vi "Get Column Info.vi"(8 "error in (no error)":errorcluster, 11 "SQLite3LV Cursor in":refnum<class "cursor.lvclass">) -> (0 "error out":errorcluster, 2 "column types":i32[](array[ring]) items=["INTEGER"=1, "FLOAT"=2, "STRING"=3, "BLOB"=4, "NULL"=5], 3 "SQLite3LV Cursor out":refnum<class "cursor.lvclass">)   [LabVIEW 2014, in "SQLite3LV.lvlib" / "cursor.lvclass"]
uses:
  cursor.lvclass
  cursor.lvclass/cursor.ctl
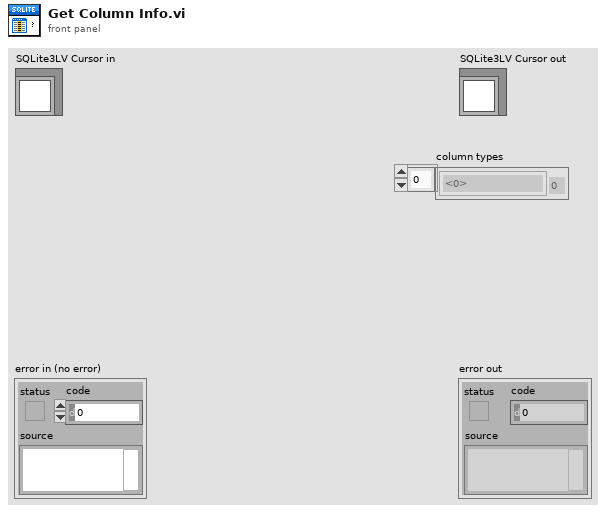
[diagram p1: front panel]
types:
  T1 = typedef "SQLite3LV.lvlib/cursor.lvclass/ctl_active_statement.ctl" = cluster{"ppStmt":i64, "column count":i32, "bind offset":i32, "bind param count":i32, "finished?":bool, "column offset":i32, "column types":i32[]}
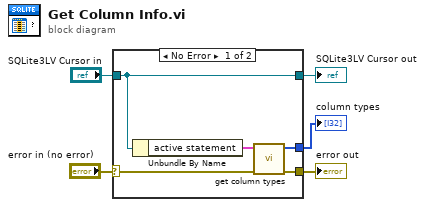
[diagram p0: block diagram]
diagram:
  n1 = case shown="No Error" "error in (no error)" {
    selector: "error in (no error)" -> [w7 w12]
    tunnel: [w6 w12] -> w4
    tunnel: [w10 w11] -> w2
    tunnel: "SQLite3LV Cursor in" -> [w10 w11]
    tunnel: [w9 _] -> w1
    frame No Error {
      n2 = Unbundle By Name(w10) -> ("active statement"=w8:T1)
      n3 = call "get column types.vi"("error in (no error)"=w7, "active statement"=w8) -> ("error out"=w6:errorcluster, "column types out"=w9:i32[])  [unwired: 8 in]
    }
    frame Error {
    }
  }
  "error out" <- w4
  "SQLite3LV Cursor out" <- w2
  "column types" <- w1
